vi "Untitled 3 (SubVI).vi"(6 "Array Index or Channel":i32, 7 "Pass?":bool, 8 "error in (no error)":errorcluster, 9 "Array Size":i32, 10 "Test Parameters":T1 {"Allowed Tolerance (%)" format="%#_4g"}, 11 "Array in":bool[](array[boolean])) -> (0 "error out":errorcluster, 1 "Boolean":bool, 2 "Record?":bool, 3 "Array out":bool[](array[boolean]), 5 "Recorded":bool[](array[boolean]))   [LabVIEW 2026]
uses:
  Test Parameters Cluster.ctl
  Processing_Engine.lvlib
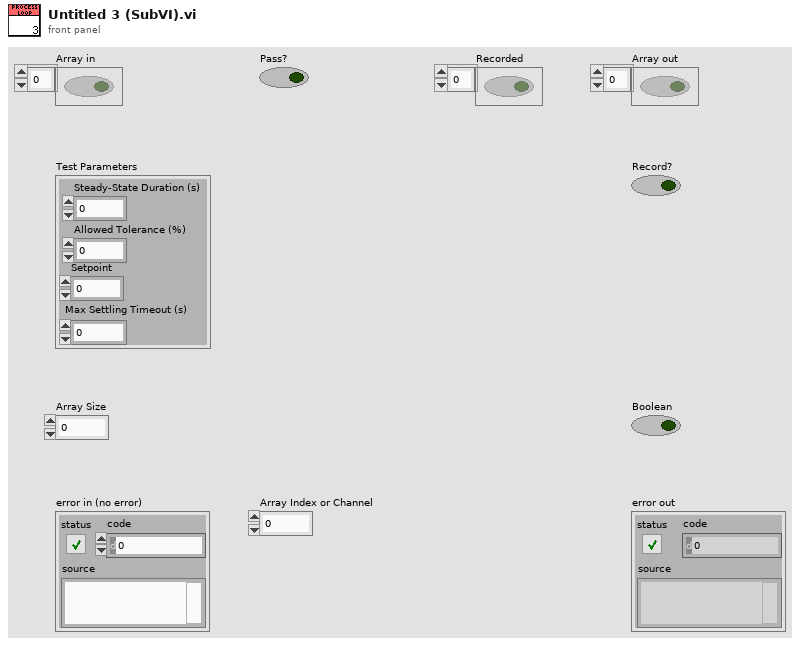
[diagram p1: front panel]
types:
  T1 = typedef "Test Parameters Cluster.ctl" = cluster{"Steady-State Duration (s)":i32, "Allowed Tolerance (%)":dbl, "Setpoint":dbl, "Max Settling Timeout (s)":i32}
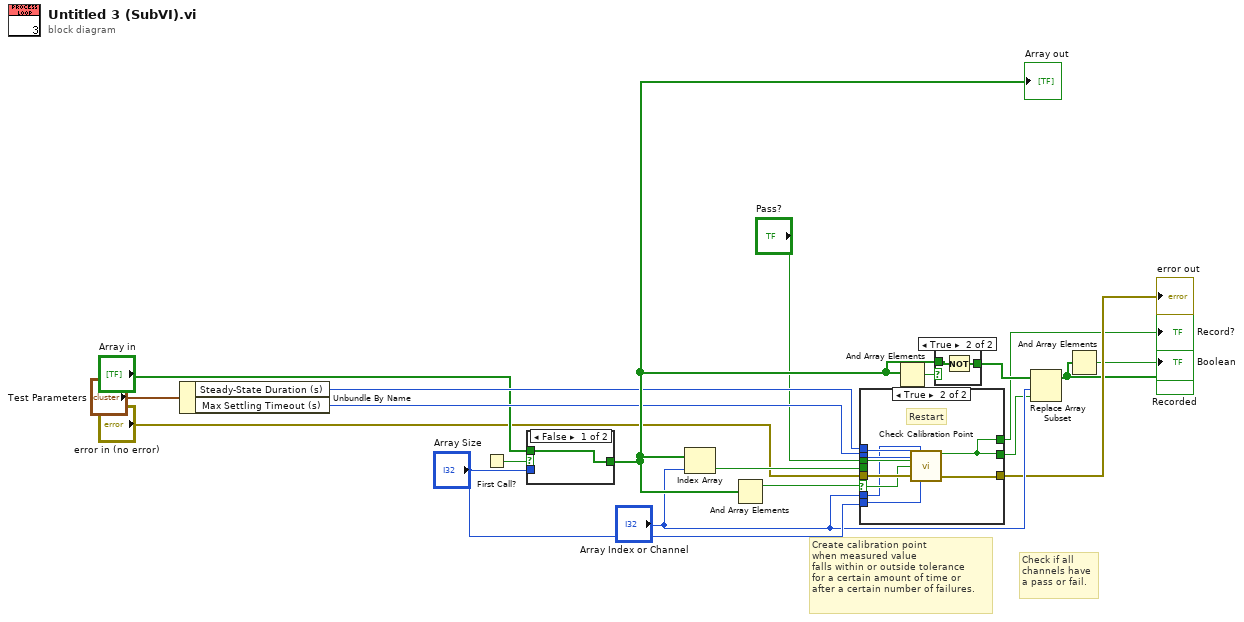
[diagram p0: block diagram]
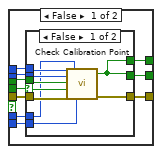
[diagram p3: hidden frame]
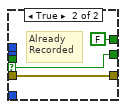
[diagram p4: hidden frame]
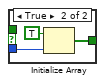
[diagram p5: hidden frame]
diagram:
  # "Create calibration point\nwhen measured value\nfalls within or outside tolerance\nfor a certain amount of time or \nafter a certain number of failures."
  # "Check if all\nchannels have\na pass or fail."
  n1 = Unbundle By Name("Test Parameters") -> ("Steady-State Duration (s)"=w12:i32, "Max Settling Timeout (s)"=w11:i32)
  n2 = First Call?() -> (First Call?: T/F=w4:bool)
  n3 = case shown="False" w4 {
    tunnel: "Array Size" -> [_ w22]
    tunnel: [w20 w21] -> w18
    tunnel: "Array in" -> [w20 _]
    frame False {
    }
    frame True {
      n4 = Initialize Array(TRUE ("Record?"), w22) -> (w21:bool[])
    }
  }
  "Array out" <- w18
  n5 = Index Array(array=w18, index="Array Index or Channel") -> (element=w6:bool)
  n6 = And Array Elements(Boolean array=w18) -> (logical AND=w7:bool)
  n7 = case shown="True" w7 {
    selector: w7 -> [_ w48]
    tunnel: "error in (no error)" -> [w33 w54]
    tunnel: [w32 w53] -> w14
    tunnel: [w31 w49] -> w8
    tunnel: "Pass?" -> [w30 w52]
    tunnel: w6 -> [w29 _]
    tunnel: w11 -> [w28 w51]
    tunnel: w12 -> [w27 w50]
    tunnel: [w26 w49] -> w13
    tunnel: "Array Index or Channel" -> [w25 w47]
    tunnel: "Array Size" -> [w24 w46]
    frame False {
      n8 = case shown="False" w29 {
        selector: w29 -> [w39 w44]
        tunnel: w33 -> [w42 w45]
        tunnel: [w41 w45] -> w32
        tunnel: [w36 w44] -> w31
        tunnel: w30 -> [w40 _]
        tunnel: w28 -> [w38 _]
        tunnel: w27 -> [w37 _]
        tunnel: [w36 FALSE] -> w26
        tunnel: w25 -> [w35 _]
        tunnel: w24 -> [w34 _]
        frame False {
          n9 = call "Check Calibration Point.vi"("Steady State Duration"=w37, "Channel"=w35, "Maximum Settling Timeout"=w38, "Pass Flag?"=w40, "Reset?"=w39, "error in (no error)"=w42, "Number of Channels"=w34) -> ("Record?"=w36:bool, "error out"=w41:errorcluster)  [unwired: 7 in]
        }
        frame True {
          # "Already\nRecorded"
        }
      }
    }
    frame True {
      # "Restart"
      n10 = call "Check Calibration Point.vi"("Steady State Duration"=w50, "Channel"=w47, "Maximum Settling Timeout"=w51, "Pass Flag?"=w52, "Reset?"=w48, "error in (no error)"=w54, "Number of Channels"=w46) -> ("Record?"=w49:bool, "error out"=w53:errorcluster)  [unwired: 7 in]
    }
  }
  "error out" <- w14
  "Record?" <- w13
  n11 = And Array Elements(Boolean array=w18) -> (logical AND=w17:bool)
  n12 = case shown="True" w17 {
    tunnel: w18 -> [w55 w57]
    tunnel: [w55 w56] -> w19
    frame False {
    }
    frame True {
      n13 = Not(x=w57) -> (.not. x?=w56:bool[])
    }
  }
  n14 = Replace Array Subset(array=w19, new element=w8, index="Array Index or Channel") -> (w3:bool[])
  "Recorded" <- w3
  n15 = And Array Elements(Boolean array=w3) -> (logical AND=→"Boolean":bool)
